vi "Do.vi"(8 "error in (no error)":errorcluster, 10 "Actor in":refnum<class "Actor.lvclass">, 11 "Result Response Msg":refnum<class "Result Response Msg.lvclass">) -> (0 "error out":errorcluster, 2 "Actor out":refnum<class "Actor.lvclass">)   [LabVIEW 2016, in "Result Response Msg.lvclass"]
doc: "This VI delivers the message to the actor by calling the appropriate method(s) on the actor."
uses:
  Result Response Msg.lvclass
  C:/github/Measure_core/Measure Object Messages/Result Reply Msg/Result Reply Msg.lvclass
  <vilib>/ActorFramework/Actor/Actor.lvclass
  Process Controller/Process Controller.lvclass
  C:/Program Files/National Instruments/LabVIEW 2016/vi.lib/ActorFramework/Actor/Actor.lvclass
  Da Base Messages/Result Reply Msg/Result Reply Msg.lvclass/Result Reply Msg.ctl
  Da Base Messages/Result Reply Msg/Read Result.vi
  Results/Acquired Result/Acquired Result.lvclass
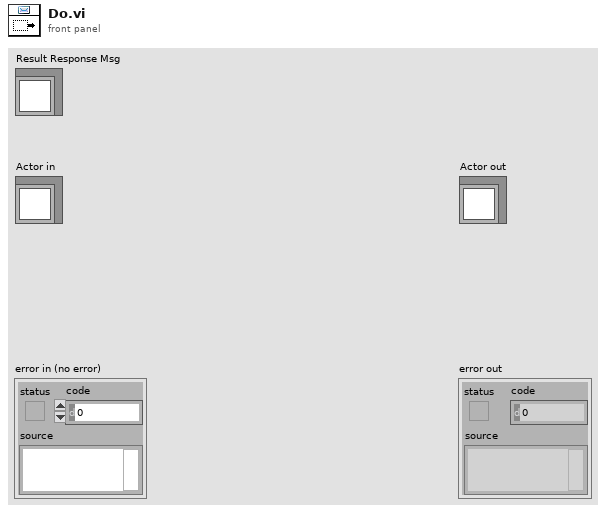
[diagram p1: front panel]
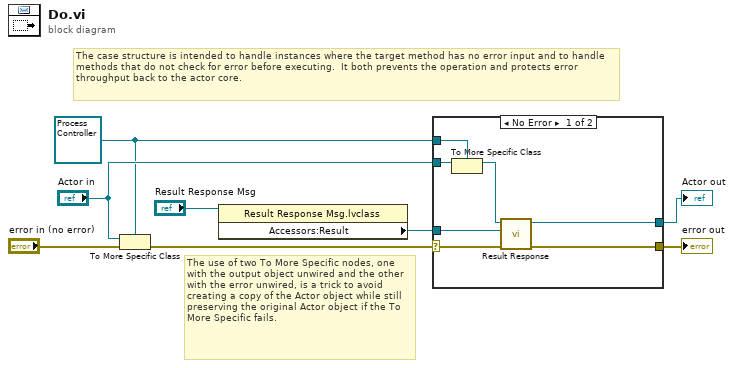
[diagram p0: block diagram]
diagram:
  w3 = refnum<class "Process Controller.lvclass"> refnum ("Actor in")
  # "The use of two To More Specific nodes, one with the output object unwired and the other with the error unwired, is a trick to avoid creating a copy of the Actor object while still preserving the original Actor object if the To More Specific fails."
  # "The case structure is intended to handle instances where the target method has no error input and to handle methods that do not check for error before executing.  It both prevents the operation and protects error throughput back to the actor core."
  n1 = To More Specific Class(target class=w3, reference="Actor in", error in="error in (no error)") -> (error out=w7:errorcluster)  [unwired: 1 out]
  n2 = property class="Result Response Msg.lvclass"(reference="Result Response Msg") -> ("Accessors:Result"=w1:refnum<class "Acquired Result.lvclass">)  [unwired: 1 in, 2 out]
  n3 = case shown="No Error" w7 {
    selector: w7 -> [w13 w17]
    tunnel: [w15 w17] -> w6
    tunnel: [w14 w16] -> w5
    tunnel: "Actor in" -> [w12 w16]
    tunnel: w3 -> [w11 _]
    tunnel: w1 -> [w9 _]
    frame No Error {
      n4 = To More Specific Class(target class=w11, reference=w12) -> (specific class reference=w10:refnum<class "Process Controller.lvclass">)  [unwired: 1 in, 1 out]
      n5 = call-dynamic "Result Response.vi"("error in (no error)"=w13, "Acquired Result"=w9, "Measure Controller in"=w10) -> ("error out"=w15:errorcluster, "Measure Controller out"=w14:refnum<class "Process Controller.lvclass">)  [unwired: 7 in]
    }
    frame Error {
      # "If type check fails, pass the original object out again."
    }
  }
  "error out" <- w6
  "Actor out" <- w5
